vi "Atto DRY Interface get Dump Pressure.vi"(8 "error in (no error)":errorcluster, 11 "DumpPressureMbar":sgl) -> (0 "error out":errorcluster, 2 "function return":i32, 3 "DumpPressureMbar out":sgl)   [LabVIEW 2016, in "attoDRYLib.lvlib"]
doc: "int32_t __cdecl AttoDRY_Interface_getDumpPressure(float *DumpPressureMbar);"
uses:
  <userlib>/attoDRYLib/attoDRYLib.lvlib
  <userlib>/attoDRYLib/attoDRYLib.dll
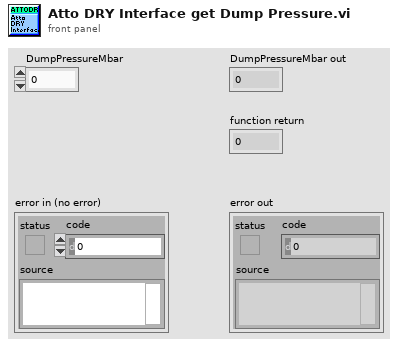
[diagram p1: front panel]
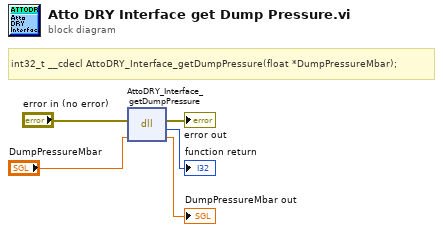
[diagram p0: block diagram]
diagram:
  # "int32_t __cdecl AttoDRY_Interface_getDumpPressure(float *DumpPressureMbar);"
  n1 = dll-call lib="C:/Program Files (x86)/National Instruments/LabVIEW 2016/user.lib/attoDRYLib/attoDRYLib.*" fn="AttoDRY_Interface_getDumpPressure"(error in="error in (no error)", "DumpPressureMbar"="DumpPressureMbar") -> (error out=→"error out":errorcluster, →"function return":i32, "DumpPressureMbar"=→"DumpPressureMbar out":sgl)  [unwired: 2 in, 1 out]
